vi "Send_active_rules_info.vi"(7 "Minimal interval, ms":u32=97, 8 "error in (no error)":errorcluster, 11 "Conditions are TRUE (active rules)":bool[](array[boolean])) -> (0 "error out":errorcluster)   [LabVIEW 2018, in "TTL IO.lvlib"]
uses:
  TTL IO.lvlib
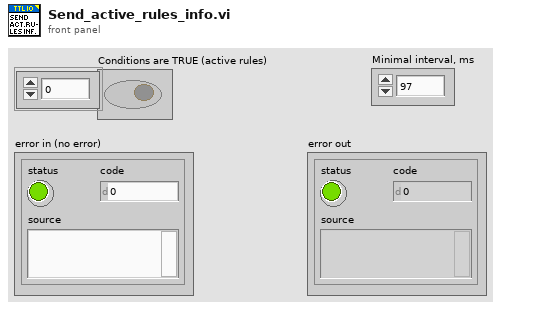
[diagram p1: front panel]
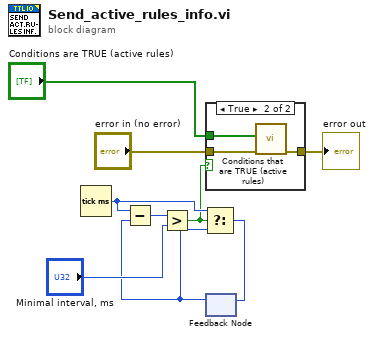
[diagram p0: block diagram]
diagram:
  n1 = Tick Count (ms)() -> (millisecond timer value=w3:u32)
  n2 = feedback #1() -> (w2:u32)  [unwired: 1 in]
  n3 = Subtract(x=w3, y=w2) -> (x-y=w9:u32)
  n4 = Greater?(x=w9, y="Minimal interval, ms") -> (0:w1:bool)
  n5 = Select(t=w3, s=w1, f=w2) -> (s? t:f=w4:u32)
  n6 = case shown="True" w1 {
    tunnel: "error in (no error)" -> [w10 w13]
    tunnel: "Conditions are TRUE (active rules)" -> [_ w12]
    tunnel: [w10 w11] -> w5
    frame False {
    }
    frame True {
      n7 = call "Conditions that are TRUE (active rules).vi"("error in (no error)"=w13, "Active rules"=w12) -> ("error out"=w11:errorcluster)  [unwired: 9 in]
    }
  }
  "error out" <- w5
  n8 = feedback-in #1(w4) -> ()
